vi "fgv_Abort Logging.vi"(8 "error in (no error)":errorcluster, 9 "Function":T1, 11 "Live Imaging?":bool) -> (0 "error out":errorcluster, 3 "Abort logging":bool)   [LabVIEW 2017]
uses:
  Typedefs/Read Write Enum.ctl
panel:
  # "SUBROUTINE"
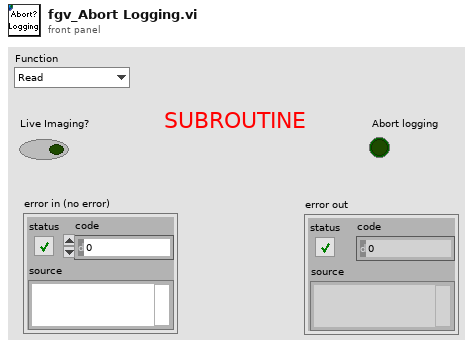
[diagram p1: front panel]
types:
  T1 = typedef "Read Write Enum.ctl" = enum16{"Read", "Write"}
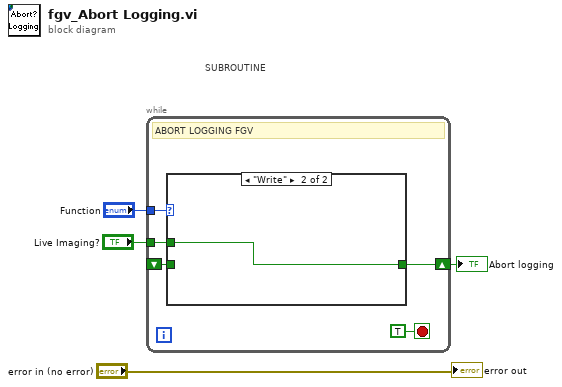
[diagram p0: block diagram]
diagram:
  # "SUBROUTINE"
  n1 = while {
    tunnel: "Function" -> [w8]
    tunnel: "Live Imaging?" -> [w7]
    shift-right: [w6] -> w2
    shift-left: _ -> [w5]
    stop <- TRUE stop-if-true
    # "ABORT LOGGING FGV"
    n2 = case shown="\"Write\"" w8 {
      tunnel: w7 -> [_ w11]
      tunnel: [w10 w11] -> w6
      tunnel: w5 -> [w10 _]
      frame "Read", Default {
      }
      frame "Write" {
      }
    }
  }
  "Abort logging" <- w2
  "error out" <- "error in (no error)"
